vi "download file.vi"(8 "error in (no error)":errorcluster, 10 "URL":string, 11 "Error message":string) -> (0 "error out":errorcluster, 3 "downloaded file":string)   [LabVIEW 2019]
uses:
  <vilib>/httpClient/LabVIEWHTTPClient.lvlib
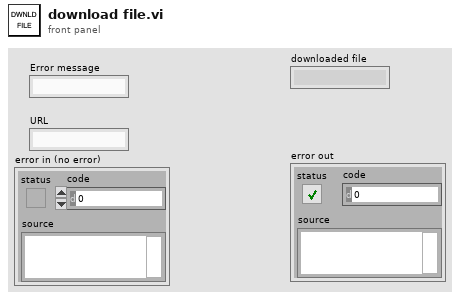
[diagram p1: front panel]
types:
  T1 = typedef "LabVIEWHTTPClient.lvlib/ClientHandle.ctl" = refnum<k1>
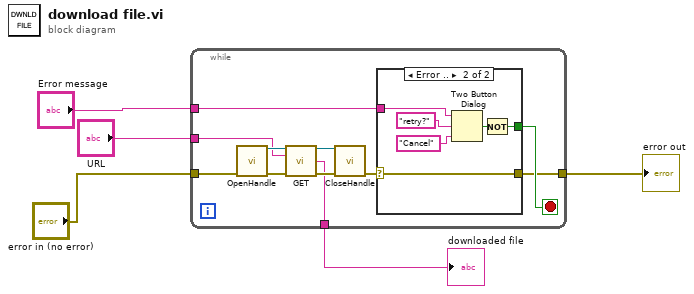
[diagram p0: block diagram]
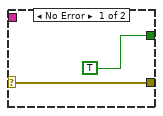
[diagram p2: hidden frame]
diagram:
  n1 = while {
    tunnel: "URL" -> [w12]
    tunnel: [w11] -> w3
    tunnel: "Error message" -> [w8]
    tunnel: "error in (no error)" -> [w7]
    tunnel: [w6] -> w1
    stop <- w9 stop-if-true
    n2 = call <vilib>:"OpenHandle.vi"("error in (no error)"=w7) -> ("client handle out"=w16:T1, "error out"=w15:errorcluster)  [unwired: 13 in]
    n3 = call <vilib>:"GET.vi"("client handle"=w16, "url"=w12, "error in (no error)"=w15) -> ("client handle out"=w13:T1, "body"=w11:string, "error out"=w14:errorcluster)  [unwired: 9 in, 1 out]
    n4 = call <vilib>:"CloseHandle.vi"("client handle"=w13, "error in (no error)"=w14) -> ("error out"=w10:errorcluster)  [unwired: 13 in]
    n5 = case shown="Error .." w10 {
      selector: w10 -> [w17 w19]
      tunnel: [TRUE w20] -> w9
      tunnel: w8 -> [_ w24]
      tunnel: [w17 w19] -> w6
      frame No Error {
      }
      frame Error {
        n6 = Two Button Dialog(message=w24, 1:"Cancel" ("F button name (\"Cancel\")"), 2:"retry?" ("T button name (\"OK\")")) -> (T button?=w22:bool)
        n7 = Not(x=w22) -> (.not. x?=w20:bool)
      }
    }
  }
  "downloaded file" <- w3
  "error out" <- w1
